vi "Lakeshore 325 Rd Wr Control Parameters.vi"(8 "error in (no error)":errorcluster, 10 "Write? (F:Read)":bool, 11 "Control Parameters":T1={"Mode"=2, "Setpoint"=0.0, "Manual Power (%)"=0.0, "Control Parameters"={"P"=0.0, "I"=0.0, "D"=0}, "Heater Range"=0, "Default Range"=0} {"Default Range" items=["Off", "Low (0.5W)", "Med (5W)", "High (50W)"]; "Heater Range" items=["Off", "Low (0.5W)", "Med (5W)", "High (50W)"]; "Manual Power (%)" format="%.3f"; "Mode" items=["Manual PID"=1, "Zone"=2, "Open Loop"=3, "AutoTune PID"=4, "AutoTune PI"=5, "AutoTune P"=6]}) -> (0 "error out":errorcluster, 3 "Control Parameters 2":T1={"Mode"=2, "Setpoint"=0.0, "Manual Power (%)"=0.0, "Control Parameters"={"P"=0.0, "I"=0.0, "D"=0}, "Heater Range"=0, "Default Range"=0} {"Default Range" items=["Off", "Low (0.5W)", "Med (5W)", "High (50W)"]; "Heater Range" items=["Off", "Low (0.5W)", "Med (5W)", "High (50W)"]; "Manual Power (%)" format="%.3f"; "Mode" items=["Manual PID"=1, "Zone"=2, "Open Loop"=3, "AutoTune PID"=4, "AutoTune PI"=5, "AutoTune P"=6]})   [LabVIEW 2024, in "Lakeshore 325.lvclass"]
uses:
  Lakeshore 325.lvclass
  Temp Control Parameters.ctl
  Temp Control.lvclass
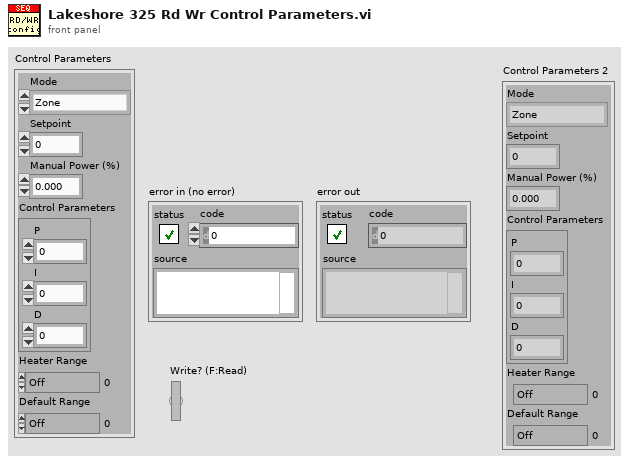
[diagram p1: front panel]
types:
  T1 = typedef "Temp Control.lvclass/Temp Control Parameters.ctl" = cluster{"Mode":u16, "Setpoint":dbl, "Manual Power (%)":dbl, "Control Parameters":cluster{"P":dbl, "I":dbl, "D":u16}, "Heater Range":u16, "Default Range":u16}
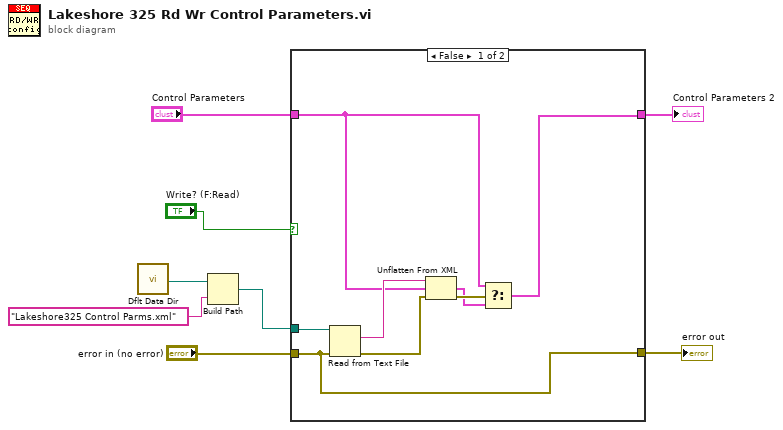
[diagram p0: block diagram]
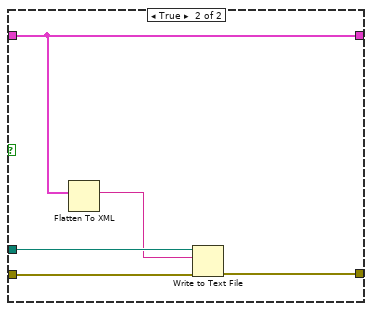
[diagram p2: hidden frame]
diagram:
  n1 = call <vilib>:"Dflt Data Dir.vi"() -> ("App:Default Data Directory"=w5:path)
  n2 = Build Path(base path=w5, name or relative path="Lakeshore325 Control Parms.xml") -> (appended path=w4:path)
  n3 = case shown="False" "Write? (F:Read)" {
    tunnel: "error in (no error)" -> [w9 w21]
    tunnel: "Control Parameters" -> [w12 w17]
    tunnel: w4 -> [w16 w20]
    tunnel: [w9 w18] -> w3
    tunnel: [w10 w17] -> w2
    frame False {
      n4 = Read from Text File(file (use dialog)=w16, error in=w9) -> (text=w15:string, error out=w14:errorcluster)  [unwired: 2 in, 2 out]
      n5 = Unflatten From XML(xml string=w15, type=w12, error in (no error)=w14) -> (value=w11:T1, error out=w13:errorcluster)
      n6 = Select(t=w12, s=w13, f=w11) -> (s? t:f=w10:T1)
    }
    frame True {
      n7 = Flatten To XML(6:w17) -> (2:w19:string)
      n8 = Write to Text File(file (use dialog)=w20, text=w19, error in=w21) -> (error out=w18:errorcluster)  [unwired: 1 in, 2 out]
    }
  }
  "error out" <- w3
  "Control Parameters 2" <- w2
